vi "WristPosition.vi"(11 "WristPositions":T1) -> (3 "WristMotorAngle":dbl)   [LabVIEW 2023]
uses:
  WristPositionsEnum.ctl
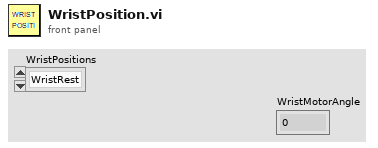
[diagram p1: front panel]
types:
  T1 = typedef "WristPositionsEnum.ctl" = enum16{"WristRest ", "WristFlat", "WristSlant"}
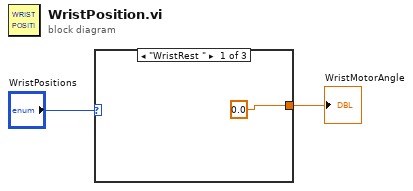
[diagram p0: block diagram]
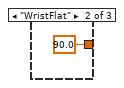
[diagram p2: hidden frame]
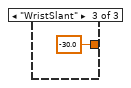
[diagram p3: hidden frame]
diagram:
  n1 = case shown="\"WristRest \"" "WristPositions" {
    tunnel: [0.0 ("WristMotorAngle") 90.0 ("WristMotorAngle") -30.0 ("WristMotorAngle")] -> w1
    frame "WristRest " {
    }
    frame "WristFlat" {
    }
    frame "WristSlant" {
    }
  }
  "WristMotorAngle" <- w1
